vi "Save File Create Folder If Needed.vi"(6 "Debug or Inv File?":T3, 7 "Prevent Startup File":bool, 8 "error in (no error)":errorcluster, 11 "File Locations In":T1) -> (0 "error out":errorcluster, 3 "File Locations Out":T1)   [LabVIEW 2016, in "Save File.lvlib"]
uses:
  Save File.lvlib
  File Setup (Public)/Type Definition/Save File DOE File Path Control.ctl
  File Setup (Public)/Type Definition/Save File DOE Data Save Filepaths.ctl
  Type Definitions/Save File Type.ctl
  File Setup.lvlib
panel:
  out "stripped path":path
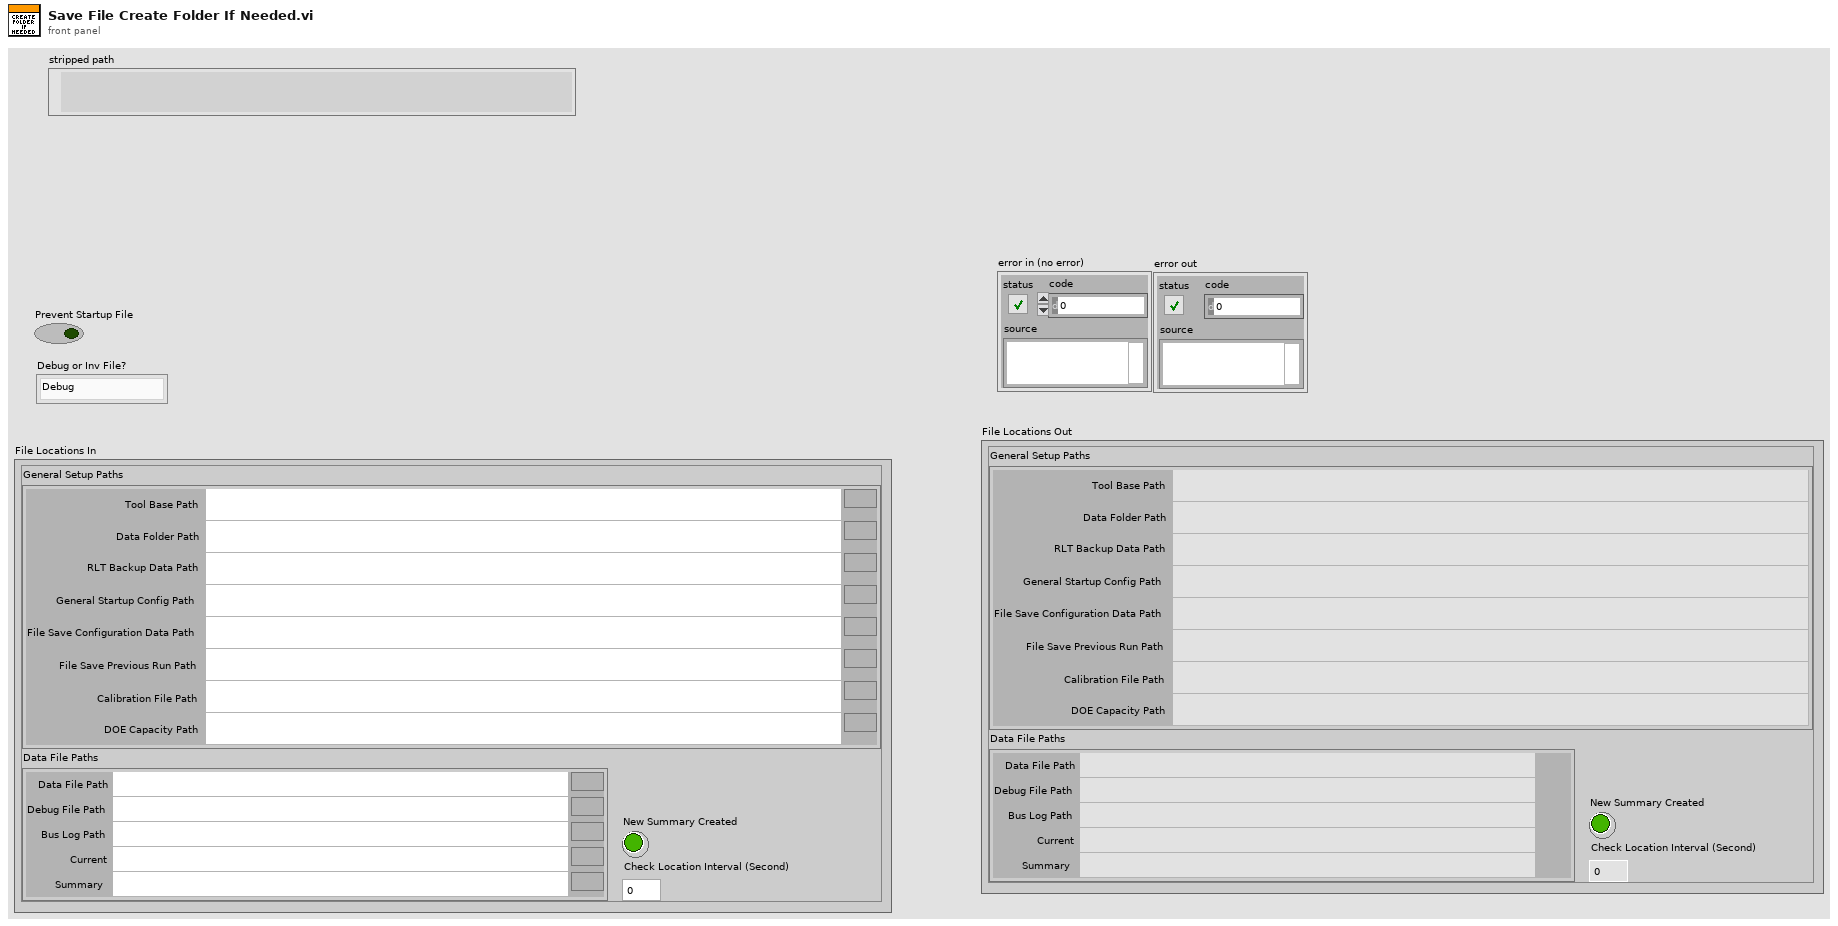
[diagram p1: front panel]
types:
  T1 = typedef "File Setup.lvlib/Save File DOE File Path Control.ctl" = cluster{"General Setup Paths":cluster{"Calibration File Path":path, "DOE Capacity Path":path, "Data Folder Path":path, "RLT Backup Data Path":path, "Tool Base Path":path, "General Startup Config Path":path, "File Save Previous Run Path":path, "File Save Configuration Data Path":path}, "Data File Paths":T2, "New Summary Created":bool, "Check Location Interval (Second)":i32}
  T2 = typedef "File Setup.lvlib/Save File DOE Data Save Filepaths.ctl" = cluster{"Data File Path":path, "Debug File Path":path, "Bus Log Path":path, "Current":path, "Summary":path}
  T3 = typedef "Save File Type.ctl" = enum16{"Debug", "Inv and MC", "Current", "Bus File"}
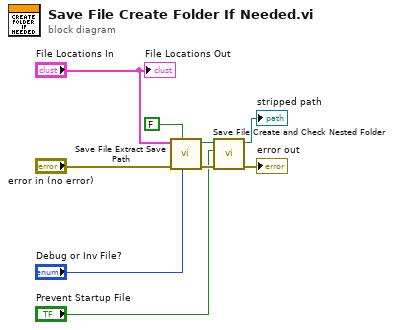
[diagram p0: block diagram]
diagram:
  n1 = call "Save File Extract Save Path.vi"("Debug or Inv File?"="Debug or Inv File?", "Extract (F)"=FALSE, "Error In"="error in (no error)", "File Locations In"="File Locations In") -> ("Error Out"=w4:errorcluster, "Extracted File Name"=w6:path)  [unwired: 5 in, 1 out]
  n2 = call "Save File Create and Check Nested Folder.vi"("error in (no error)"=w4, "Prevent Startup File"="Prevent Startup File", "Extracted File Name"=w6) -> ("error out"=→"error out":errorcluster, "Base Path"=→"stripped path":path)  [unwired: 6 in, 1 out]
  "File Locations Out" <- "File Locations In"
